vi "Query TEC Temperature.vi"(8 "error in (no error)":errorcluster, 11 "VISA resource name":refnum<visa-resource-name>) -> (0 "error out":errorcluster, 2 "TEC Temperature (°C)":dbl, 3 "VISA resource name out":refnum<visa-resource-name>)   [LabVIEW 2013, in "Ocean Optics 2000 4000.lvlib"]
doc: "Returns the instrument's Thermo Electric Cooling(TEC) Temperature.\n\n<b>Note:</b>\nOnly applicable on NIRQuest512, NIRQuest256 and QE65000."
uses:
  <instrlib>/Ocean Optics 2000 4000/Ocean Optics 2000 4000.lvlib
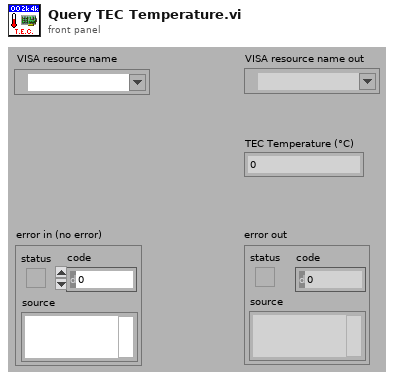
[diagram p1: front panel]
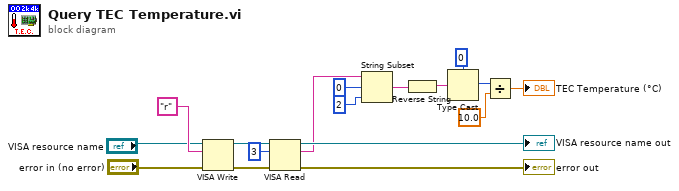
[diagram p0: block diagram]
diagram:
  n1 = VISA Write(VISA resource name="VISA resource name", write buffer="r", error in (no error)="error in (no error)") -> (VISA resource name out=w15:refnum<visa-resource-name>, error out=w16:errorcluster)  [unwired: 1 out]
  n2 = VISA Read(VISA resource name=w15, byte count=u32 3, error in (no error)=w16) -> (VISA resource name out=→"VISA resource name out":refnum<visa-resource-name>, read buffer=w8:string, error out=→"error out":errorcluster)  [unwired: 1 out]
  n3 = String Subset(string=w8, offset (0)=0, length (rest)=2 ("length (rest)")) -> (substring=w7:string)
  n4 = Reverse String(1:w7) -> (0:w6:string)
  n5 = Type Cast(type=i16 0, x=w6) -> (*(type *) &x=w4:i16)
  n6 = Divide(x=w4, y=10.0) -> (x/y=→"TEC Temperature (°C)":dbl)
